vi "Read piece type.vi"(11 "Pawn in":refnum<class "Pawn.lvclass">) -> (2 "Piece type":T1)   [LabVIEW 2016, in "Chesslib.lvlib" / "Pawn.lvclass"]
uses:
  Pawn.lvclass
  typedef/Piece type.ctl
  Chesslib.lvlib
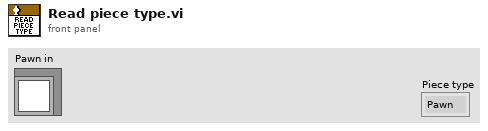
[diagram p1: front panel]
types:
  T1 = typedef "Chesslib.lvlib/Piece type.ctl" = enum16{"Pawn", "Bishop", "Knight", "Rook", "Queen", "King"}
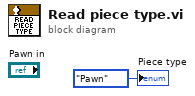
[diagram p0: block diagram]
diagram:
  "Piece type" <- Piece_type."Pawn" ("Piece type")
